vi "predict_carriers.vi"(6 "Modulation info":T1={"Fs full"=0.0, "Fs high"=0.0, "Fs low"=0.0, "Read size"=0, "FFT size low"=5000, "df low"=5000.0, "High carriers"=[], "Low carriers"=[], "Hi channels at low"=[7]} {"Hi channels at low" min=0 step=1; "Low carriers" format="%#_6p"; "High carriers" format="%#_6p"}, 7 "Low rate block start":bool, 8 "Low carrier amplitudes":cdb[](array[numeric]), 9 "KF in":T2 {"K" format="%#_3g"; "y lim" format="%#_3g"; "x lim" format="%#_3g"; "P" format="%#_3g"; "H" format="%#_3g"; "x" format="%#_3g"; "Q" format="%#_3g"; "R" format="%#_3g"; "B" format="%#_3g"; "A" format="%#_3g"}, 10 "Reset":bool, 11 "Config":T4={"I/O"={"Format"={"Rate"=4, "Bits"=32, "Channels"=2}, "card #"=1, "# buffers"=96000}, "High rate STFT"={"Win param"=101.5, "Window type"=61, "Win order"=2, "DFT size"=64, "Channels"=[7], "Oversample"=64}, "Low rate STFT"={"Win param"=120.0, "Window type"=61, "Win order"=8, "DFT size"=64, "Channels"=[7], "Oversample"=64}, "Filtering"={"Hum"={"Frequency"=0.0, "Tc"=0.0, "Limit"=101.5, "FFT filter"=FALSE, "Detrend mode"=enum."Robust linear", "Enable"=FALSE}, "Kalman"={"Process noise"=101.5, "Measure noise"=101.5, "Unlock m noise"=101.5, "Mode"=enum."FFT"}, "Distortion"={"LF cut"=101.5, "Tc"=3.0, "Limit"=101.5, "FFT filter"=FALSE, "Detrend mode"=enum."Robust linear", "Enable"=FALSE}, "Lowpass"={"Frequency"=0.0, "Order"=0, "Enable"=FALSE}, "Impulse"={"Win order"=102, "Locked limit"=101.5, "Locked count"=102, "Threshold Tc"=101.5, "Thresh sigmas"=101.5, "Thresh min"=101.5, "After"=0, "Detrend"=FALSE, "Enable"=FALSE}}} {"Filtering"."Impulse"."Thresh min" format="%#_3p"; "Filtering"."Impulse"."Threshold Tc" format="%#_3p"; "Filtering"."Impulse"."Locked limit" format="%#_3p"; "Filtering"."Impulse"."Thresh sigmas" format="%#_3p"; "Filtering"."Lowpass"."Frequency" format="%#_4p"; "Filtering"."Distortion"."Limit" format="%#_3p"; "Filtering"."Distortion"."LF cut" format="%#_3p"; "Filtering"."Kalman"."Unlock m noise" format="%#_3p"; "Filtering"."Kalman"."Measure noise" format="%#_3p"; "Filtering"."Kalman"."Process noise" format="%#_3p"; "Filtering"."Hum"."Limit" format="%#_3p"; "Filtering"."Hum"."Frequency" format="%#_4p"; "Low rate STFT"."Oversample" min=1 step=1; "Low rate STFT"."Channels" min=0 step=1; "Low rate STFT"."DFT size" min=1 step=1; "Low rate STFT"."Window type" items=["Rectangle"=0, "Hanning"=1, "Hamming"=2, "Blackman-Harris"=3, "Exact Blackman"=4, "Blackman"=5, "Flat Top"=6, "4 Term B-Harris "=7, "7 Term B-Harris"=8, "Low Sidelobe"=9, "Blackman Nuttall"=11, "Triangle"=30, "Bartlett-Hanning"=31, "Bohman"=32, "Parzen"=33, "Welch"=34, "Kaiser"=60, "Dolph-Chebyshev"=61, "Gaussian"=62]; "High rate STFT"."Oversample" min=1 step=1; "High rate STFT"."Channels" min=0 step=1; "High rate STFT"."DFT size" min=1 step=1; "High rate STFT"."Window type" items=["Rectangle"=0, "Hanning"=1, "Hamming"=2, "Blackman-Harris"=3, "Exact Blackman"=4, "Blackman"=5, "Flat Top"=6, "4 Term B-Harris "=7, "7 Term B-Harris"=8, "Low Sidelobe"=9, "Blackman Nuttall"=11, "Triangle"=30, "Bartlett-Hanning"=31, "Bohman"=32, "Parzen"=33, "Welch"=34, "Kaiser"=60, "Dolph-Chebyshev"=61, "Gaussian"=62]}) -> (2 "KF out":T2 {"K" format="%#_3g"; "y lim" format="%#_3g"; "x lim" format="%#_3g"; "P" format="%#_3g"; "H" format="%#_3g"; "x" format="%#_3g"; "Q" format="%#_3g"; "R" format="%#_3g"; "B" format="%#_3g"; "A" format="%#_3g"}, 3 "Predicted carriers":dbl[](graph))   [LabVIEW 2014]
uses:
  utilities/labview/kalman_filter.ctl
  <vilib>/Analysis/Matrix/Datatypes/RealMatrix.ctl
  ilemt_config.ctl
  io_config.ctl
  stft_params.ctl
  <vilib>/Analysis/4window.llb/windowTd.ctl
  filter_params.ctl
  detrend_mode.ctl
  modulation_info.ctl
  <vilib>/Analysis/2dsp.llb/Inverse Real FFT.vi
  <vilib>/Analysis/Matrix/NI_Matrix.lvlib
  <vilib>/Analysis/NI_AALPro.lvlib
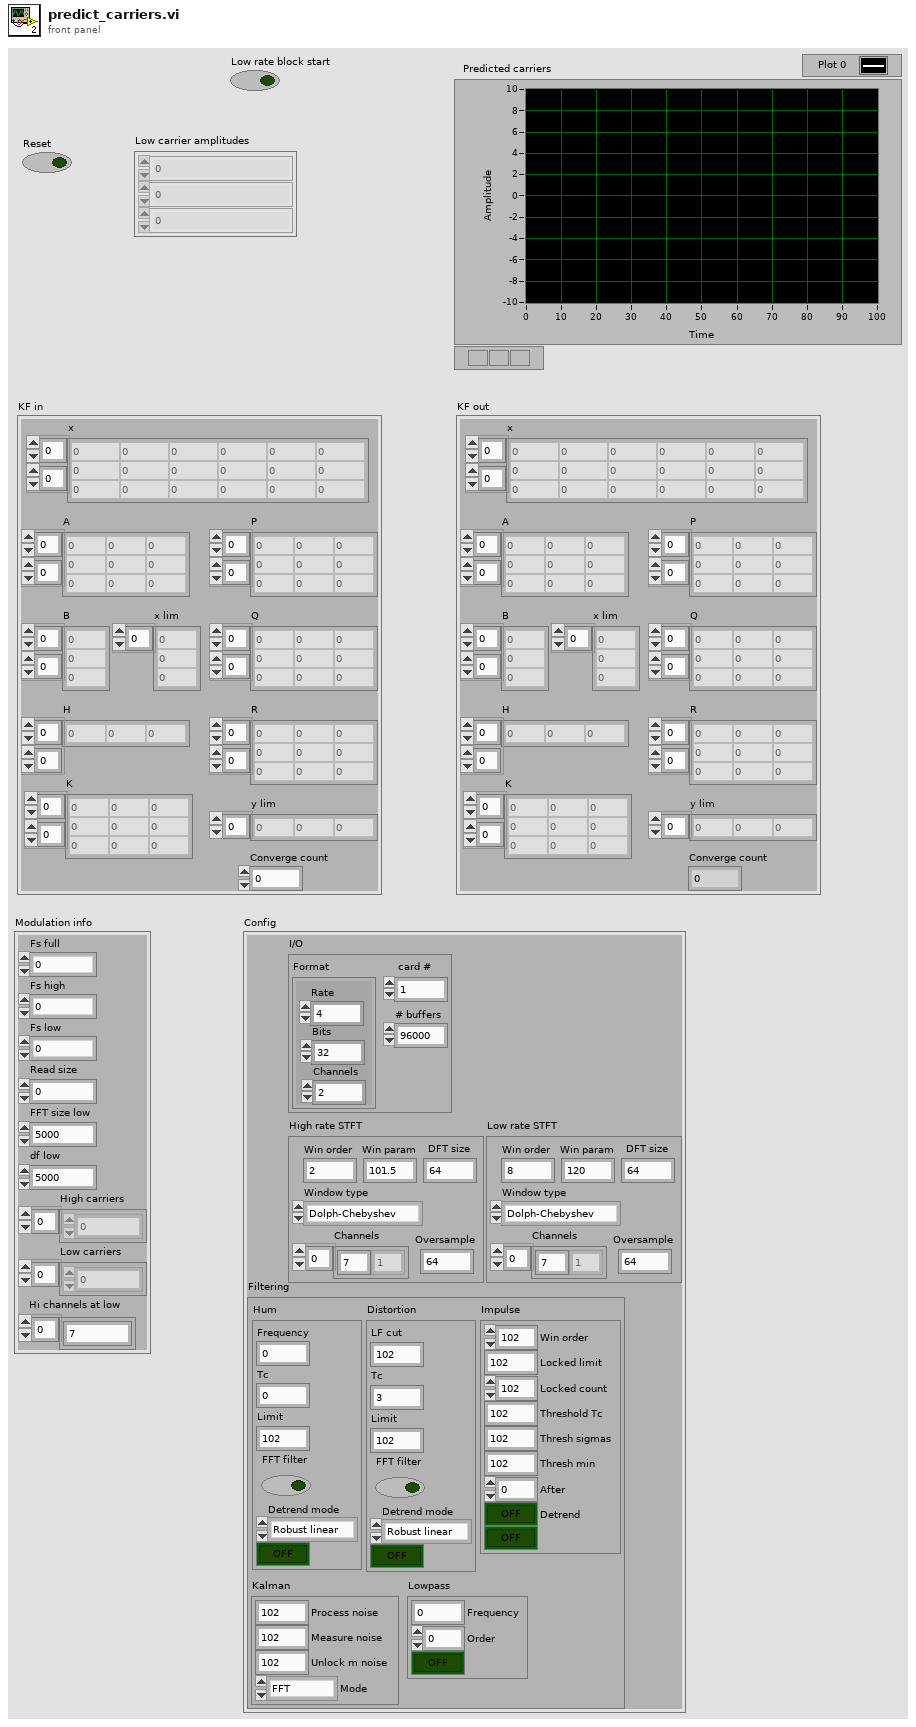
[diagram p1: front panel]
types:
  T1 = typedef "modulation_info.ctl" = cluster{"Fs full":dbl, "Fs high":dbl, "Fs low":dbl, "Read size":i32, "FFT size low":i32, "df low":dbl, "High carriers":dbl[], "Low carriers":dbl[], "Hi channels at low":i32[]}
  T2 = typedef "kalman_filter.ctl" = cluster{"A":T3, "B":T3, "H":T3, "Q":T3, "R":T3, "x":T3, "P":T3, "x lim":dbl[], "y lim":dbl[], "K":T3, "Converge count":i32}
  T3 = typedef "NI_Matrix.lvlib/RealMatrix.ctl" = dbl[][]
  T4 = typedef "ilemt_config.ctl" = cluster{"I/O":T5, "High rate STFT":T6, "Low rate STFT":T6, "Filtering":T8}
  T5 = typedef "io_config.ctl" = cluster{"Format":cluster{"Rate":i32, "Bits":i32, "Channels":u32}, "card #":u32, "# buffers":i32}
  T6 = typedef "stft_params.ctl" = cluster{"Win param":dbl, "Window type":T7, "Win order":i32, "DFT size":i32, "Channels":i32[], "Oversample":i32}
  T7 = typedef "NI_AALPro.lvlib/windowTd.ctl" = u32
  T8 = typedef "filter_params.ctl" = cluster{"Hum":cluster{"Frequency":dbl, "Tc":dbl, "Limit":dbl, "FFT filter":bool, "Detrend mode":T9, "Enable":bool}, "Kalman":cluster{"Process noise":dbl, "Measure noise":dbl, "Unlock m noise":dbl, "Mode":enum16{"FFT", "KF demod"}}, "Distortion":cluster{"LF cut":dbl, "Tc":dbl, "Limit":dbl, "FFT filter":bool, "Detrend mode":T9, "Enable":bool}, "Lowpass":cluster{"Frequency":dbl, "Order":i32, "Enable":bool}, "Impulse":cluster{"Win order":i32, "Locked limit":dbl, "Locked count":i32, "Threshold Tc":dbl, "Thresh sigmas":dbl, "Thresh min":dbl, "After":i32, "Detrend":bool, "Enable":bool}}
  T9 = typedef "detrend_mode.ctl" = enum16{"Zero mean", "Linear", "Robust linear"}
  T10 = cluster{"Process noise":dbl, "Measure noise":dbl, "Unlock m noise":dbl, "Mode":enum16{"FFT", "KF demod"}}
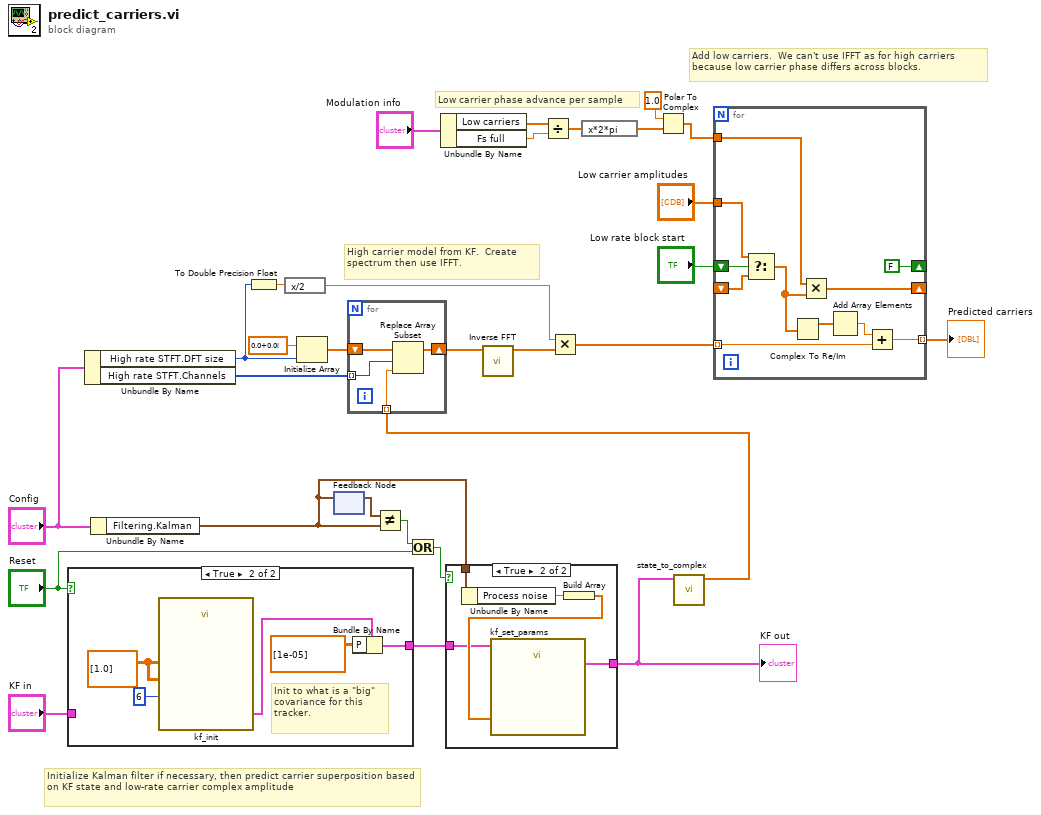
[diagram p0: block diagram]
diagram:
  # "Add low carriers.  We can't use IFFT as for high carriers because low carrier phase differs across blocks."
  # "High carrier model from KF.  Create spectrum then use IFFT."
  # "Initialize Kalman filter if necessary, then predict carrier superposition based on KF state and low-rate carrier complex amplitude"
  # "Low carrier phase advance per sample"
  n1 = case shown="True" "Reset" {
    tunnel: [w30 w31] -> w27
    tunnel: "KF in" -> [w30 _]
    frame False {
    }
    frame True {
      w34 = T3 [[1.0]] ("A")
      # "Init to what is a \"big\" covariance for this tracker."
      n2 = call "kf_init.vi"("A"=w34, "H"=w34, "x columns"=6) -> ("KF out"=w33:T2)  [unwired: 12 in]
      n3 = Bundle By Name(cluster=w33, "P"=T3 [[1e-05]] ("A")) -> (w31:T2)
    }
  }
  n4 = Unbundle By Name("Config") -> ("High rate STFT.DFT size"=w4:i32, "High rate STFT.Channels"=w21:i32[])
  n5 = Unbundle By Name("Config") -> ("Filtering.Kalman"=w29:T10)
  n6 = To Double Precision Float(number=w4) -> (double precision float=w10:dbl)
  n7 = expression code="x/2"(w10) -> (w8:dbl)
  n8 = Initialize Array(cdb 0.0+0.0i ("element"), w4) -> (w22:cdb[])
  n9 = feedback #1() -> (w26:T10)  [unwired: 1 in]
  n10 = feedback-in #1(w29) -> ()
  n11 = Not Equal?(x=w26, y=w29) -> (x != y?=w5:bool)
  n12 = Or(x=w5, y="Reset") -> (x .or. y?=w6:bool)
  n13 = Unbundle By Name("Modulation info") -> ("Low carriers"=w15:dbl[], "Fs full"=w14:dbl)
  n14 = case shown="True" w6 {
    tunnel: w27 -> [w36 w38]
    tunnel: w29 -> [_ w41]
    tunnel: [w36 w37] -> w28
    frame False {
    }
    frame True {
      n15 = Unbundle By Name(w41) -> ("Process noise"=w40:dbl)
      n16 = Build Array(w40) -> (w39:dbl[])
      n17 = call "kf_set_params.vi"("KF in"=w38, "Process noise"=w39) -> ("KF out"=w37:T2)  [unwired: 17 in]
    }
  }
  "KF out" <- w28
  n18 = Divide(x=w15, y=w14) -> (x/y=w13:dbl[])
  n19 = expression code="x*2*pi"(w13) -> (w12:dbl[])
  n20 = Polar To Complex(1:w12, 2:1.0 ("Fs full")) -> (0:w3:cdb[])
  n21 = call "state_to_complex.vi"("KF in"=w28) -> ("Amplitudes"=w20:cdb[])  [unwired: 10 in]
  n22 = for {
    tunnel: w21 -> [w43] mode=indexing
    tunnel: w20 -> [w44] mode=indexing
    shift-right: [w42] -> w19
    shift-left: w22 -> [w45]
    n23 = Replace Array Subset(array=w45, new element=w44, index=w43) -> (w42:cdb[])
  }
  n24 = call-poly <vilib>:"Inverse FFT.vi"("FFT {X}"=w19) -> ("X"=w9:dbl[])  [unwired: 9 in, 1 out]
  n25 = Multiply(x=w8, y=w9) -> (x*y=w2:dbl[])
  n26 = for {
    tunnel: w2 -> [w53] mode=indexing
    shift-right: [w52] -> _
    shift-left: _ -> [w54]
    tunnel: "Low carrier amplitudes" -> [w55]
    tunnel: w3 -> [w50]
    shift-right: [FALSE ("Low rate block start")] -> _
    shift-left: "Low rate block start" -> [w56]
    tunnel: [w46] -> w1 mode=indexing
    n27 = Select(t=w55, s=w56, f=w54) -> (s? t:f=w51:cdb[])
    n28 = Complex To Re/Im(x + iy=w51) -> (x=w48:dbl[])  [unwired: 1 out]
    n29 = Multiply(x=w50, y=w51) -> (x*y=w52:cdb[])
    n30 = Add Array Elements(numeric array=w48) -> (sum=w47:dbl)
    n31 = Add(x=w47, y=w53) -> (x+y=w46:dbl)
  }
  "Predicted carriers" <- w1
